vi "Update Sensor Number.vi"(8 "error in (no error)":errorcluster, 11 "Main Model in":refnum<class "Main Model.lvclass">) -> (0 "error out":errorcluster, 3 "Main Model out":refnum<class "Main Model.lvclass">)   [LabVIEW 2013, in "Main Model.lvlib" / "Main Model.lvclass"]
uses:
  Main Model.lvclass
  Main Model.lvclass/Main Model.ctl
  <vilib>/ActorFrameworkMVC/View Observer/View Registry/View Registry.lvclass/View Registry.ctl
  Main Model Messages/Sensor Number Msg/Sensor Number Msg.lvclass
  <vilib>/ActorFrameworkMVC/View Observer/Data Message/Data Message.lvclass
  <vilib>/ActorFrameworkMVC/View Observer/View Registry/View Registry.lvclass
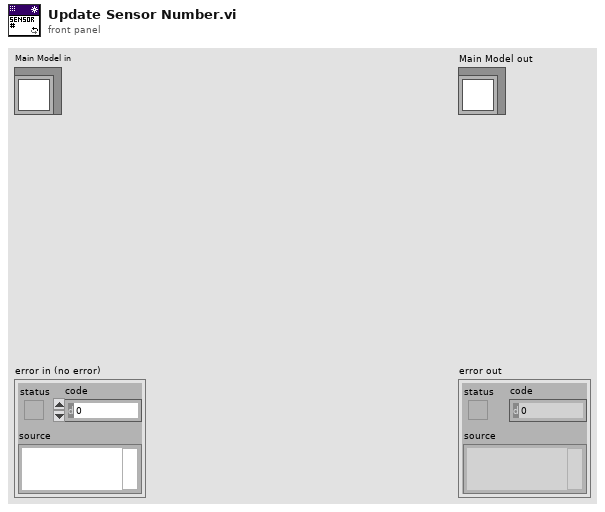
[diagram p1: front panel]
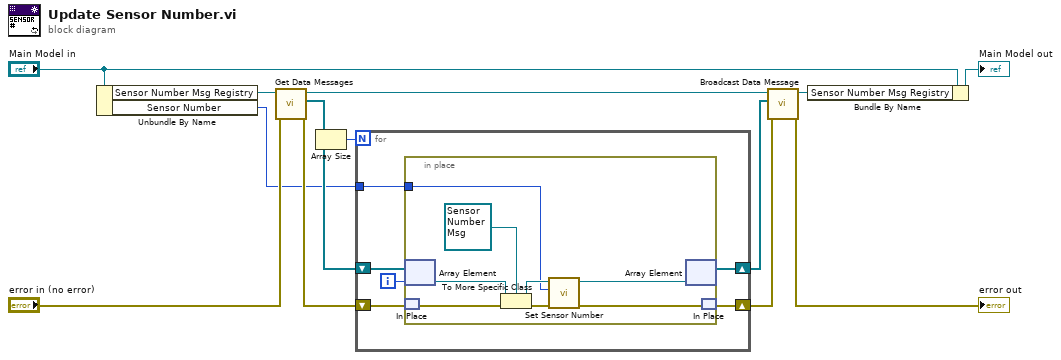
[diagram p0: block diagram]
diagram:
  n1 = Unbundle By Name("Main Model in") -> ("Sensor Number Msg Registry"=w9:refnum<class "View Registry.lvclass">, "Sensor Number"=w4:i32)
  n2 = call <vilib>:"Get Data Messages.vi"("error in (no error)"="error in (no error)", "View Registry in"=w9) -> ("error out"=w5:errorcluster, "Data Messages"=w6:refnum<class "Data Message.lvclass">[], "View Registry out"=w8:refnum<class "View Registry.lvclass">)  [unwired: 7 in]
  n3 = Array Size(array=w6) -> (size(s)=w7:i32)
  n4 = for {
    N: w7 -> [_]
    shift-right: [w18] -> w3
    shift-left: w6 -> [w19]
    shift-right: [w15] -> w2
    shift-left: w5 -> [w17]
    tunnel: w4 -> [w16]
    i -> [w14]
    n5 = in-place {
      in-place-border: w16 -> [w20]
      n6 = in-place-array #1(w19, w14) -> (w25:refnum<class "Data Message.lvclass">)
      n7 = in-place-match #2(w17) -> (w27:errorcluster)
      n8 = To More Specific Class(target class=refnum<class "Sensor Number Msg.lvclass"> refnum ("Main Model.lvlib:Sensor Number Msg.lvclass"), reference=w25, error in=w27) -> (specific class reference=w21:refnum<class "Sensor Number Msg.lvclass">, error out=w24:errorcluster)
      n9 = call-dynamic "Set Sensor Number.vi"("error in (no error)"=w24, "Sensor Number"=w20, "Project Number Msg in"=w21) -> ("error out"=w23:errorcluster, "Project Number Msg out"=w22:refnum<class "Sensor Number Msg.lvclass">)  [unwired: 7 in]
      n10 = in-place-array #1(w22) -> (w18:refnum<class "Data Message.lvclass">[])  [unwired: 1 out]
      n11 = in-place-match #2(w23) -> (w15:errorcluster)
    }
  }
  n12 = call <vilib>:"Broadcast Data Message.vi"("error in (no error)"=w2, "Data Messages"=w3, "View Registry in"=w8) -> ("error out"=→"error out":errorcluster, "View Registry out"=w1:refnum<class "View Registry.lvclass">)  [unwired: 7 in]
  n13 = Bundle By Name(cluster="Main Model in", "Sensor Number Msg Registry"=w1) -> (→"Main Model out":refnum<class "Main Model.lvclass">)
